vi "Best_n_routine_PN.vi"(3 "fixed n":dbl=0.4, 4 "variable n?":bool=TRUE, 5 "U":dbl[](array[numeric])=[1.9700640366, 2.9544254558, 3.9511341522, 4.988746499, 5.9653548413, 6.955762857, 7.9505145639, 8.9534679688, 9.9841669593, 10.940163718], 6 "E^2":dbl[](array[numeric])=[2.545899323848856, 2.7039683334539926, 2.834095502347166, 2.9505738427182537, 3.0478567682958038, 3.136700737890616, 3.218281943968314, 3.2949717775853564, 3.3680504701927467, 3.4322041581183096]) -> (0 "n":dbl=0.3999859587965401 format="%#_18g", 1 "B":dbl=0.6862228365898919 format="%#_18g", 2 "A":dbl=1.6456605879472355 format="%#_18g")   [LabVIEW 2010]
uses:
  <vilib>/Analysis/7linalg.llb/Solve Linear Equations (single right hand).vi
  <vilib>/Analysis/baseanly.llb/Real A x B.vi
  <vilib>/Analysis/7linalg.llb/Solve Linear Eqs (General).vi
  <vilib>/Analysis/7linalg.llb/Solve Linear Eqs (Gen, single right hand).vi
  <vilib>/Analysis/Matrix/Numeric/Conversions/Array To Matrix - RA2.vi
  <vilib>/Analysis/7linalg.llb/Real Transpose Matrix.vi
  <vilib>/Analysis/baseanly.llb/Real Inverse Matrix.vi
  <vilib>/Analysis/baseanly.llb/A x Vector.vi
  Globals/Dynamic_call_global.ph.vi
  <vilib>/Analysis/NI_AALPro.lvlib
  <vilib>/Analysis/NI_AALBase.lvlib
  <vilib>/Analysis/Matrix/NI_Matrix.lvlib
panel:
  in  "dn":dbl=0.0001
  in  "nmin":dbl=0.2
  in  "nmax":dbl=0.8
  in  "output RMS err?":bool=TRUE
  out "RMS err in U (m/s)":dbl=0.002670941583711803 format="%#_3f"
  out "abs rel. err.":dbl[](array[numeric])=[3.983055063353366e-13, 8.213953245912097e-13, 5.386158518578956e-13] format="%#.6e"
  out "NLR against data":cluster{dbl[], "U":dbl[]}[](graph)=[{[0.1, 0.122, 0.14884, 0.1815848, 0.221533456, 0.27027081632, 0.3297303959104, 0.402271083010688, 0.49077072127303933, 0.598740279953108, 0.7304631415427917, 0.8911650326822058, 1.087221339872291, 1.326410034644195, 1.6182202422659178, 1.9742286955644197, 2.408559008588592, 2.9384419904780823, 3.5848992283832604, 4.3735770586275775, 5.335764011525645, 6.509632094061287, 7.94175115475477, 9.688936408800819, 11.820502418736998, 14.421012950859138, 17.593635800048148, 21.46423567605874, 26.18636752479166, 31.947368380245823], "U"=[1.918859652465371, 1.9414767700229, 1.9659662732253556, 1.992483169800597, 2.021195299980173, 2.052284398853782, 2.0859472466720375, 2.1223969143784562, 2.161864112254325, 2.204598650212778, 2.2508710189851024, 2.3009741022074746, 2.3552250302448847, 2.413967187486141, 2.477572385815227, 2.5464432180161425, 2.6210156060072305, 2.7017615600341864, 2.7891921662862273, 2.8838608218457082, 2.9863667374469767, 3.097358730215403, 3.2175393303929196, 3.34766922804385, 3.488572087886694, 3.6411397627276374, 3.8063379384945, 3.985212246601707, 4.178894882334845, 4.388611771146246]}, {[1.9700640366, 2.9544254558, 3.9511341522, 4.988746499, 5.9653548413, 6.955762857, 7.9505145639, 8.9534679688, 9.9841669593, 10.940163718], "U"=[2.545899323848856, 2.7039683334539926, 2.834095502347166, 2.9505738427182537, 3.0478567682958038, 3.136700737890616, 3.218281943968314, 3.2949717775853564, 3.3680504701927467, 3.4322041581183096]}]
  in  "n0":dbl=1.0
  in  "B0":dbl=2.0
  in  "A0":dbl=10.0
  in  "show iters\ngraphically":bool
  in  "tol.":dbl=1e-12
  in  "max. iter":i32=1000
  in  "retardation":dbl=0.5
  out "Iterations":i32=47
  # "Linearise by Taylor series up to first order."
  # "if variable n is false, then this value is used for n"
  # "for coersion"
  # "r is the retardation parameter 0...1"
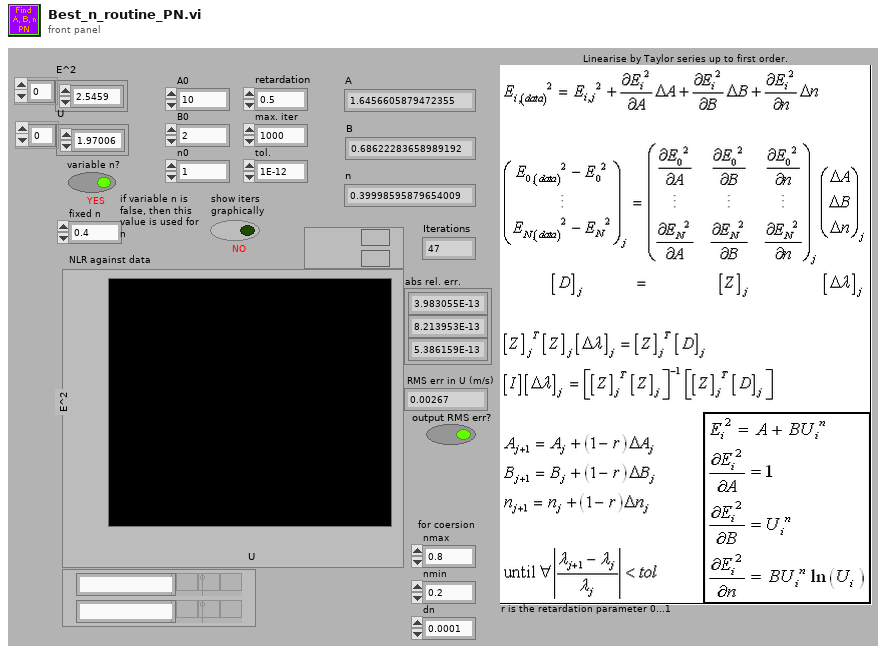
[diagram p1: front panel]
types:
  T1 = typedef "NI_Matrix.lvlib/RealMatrix.ctl" = dbl[][]
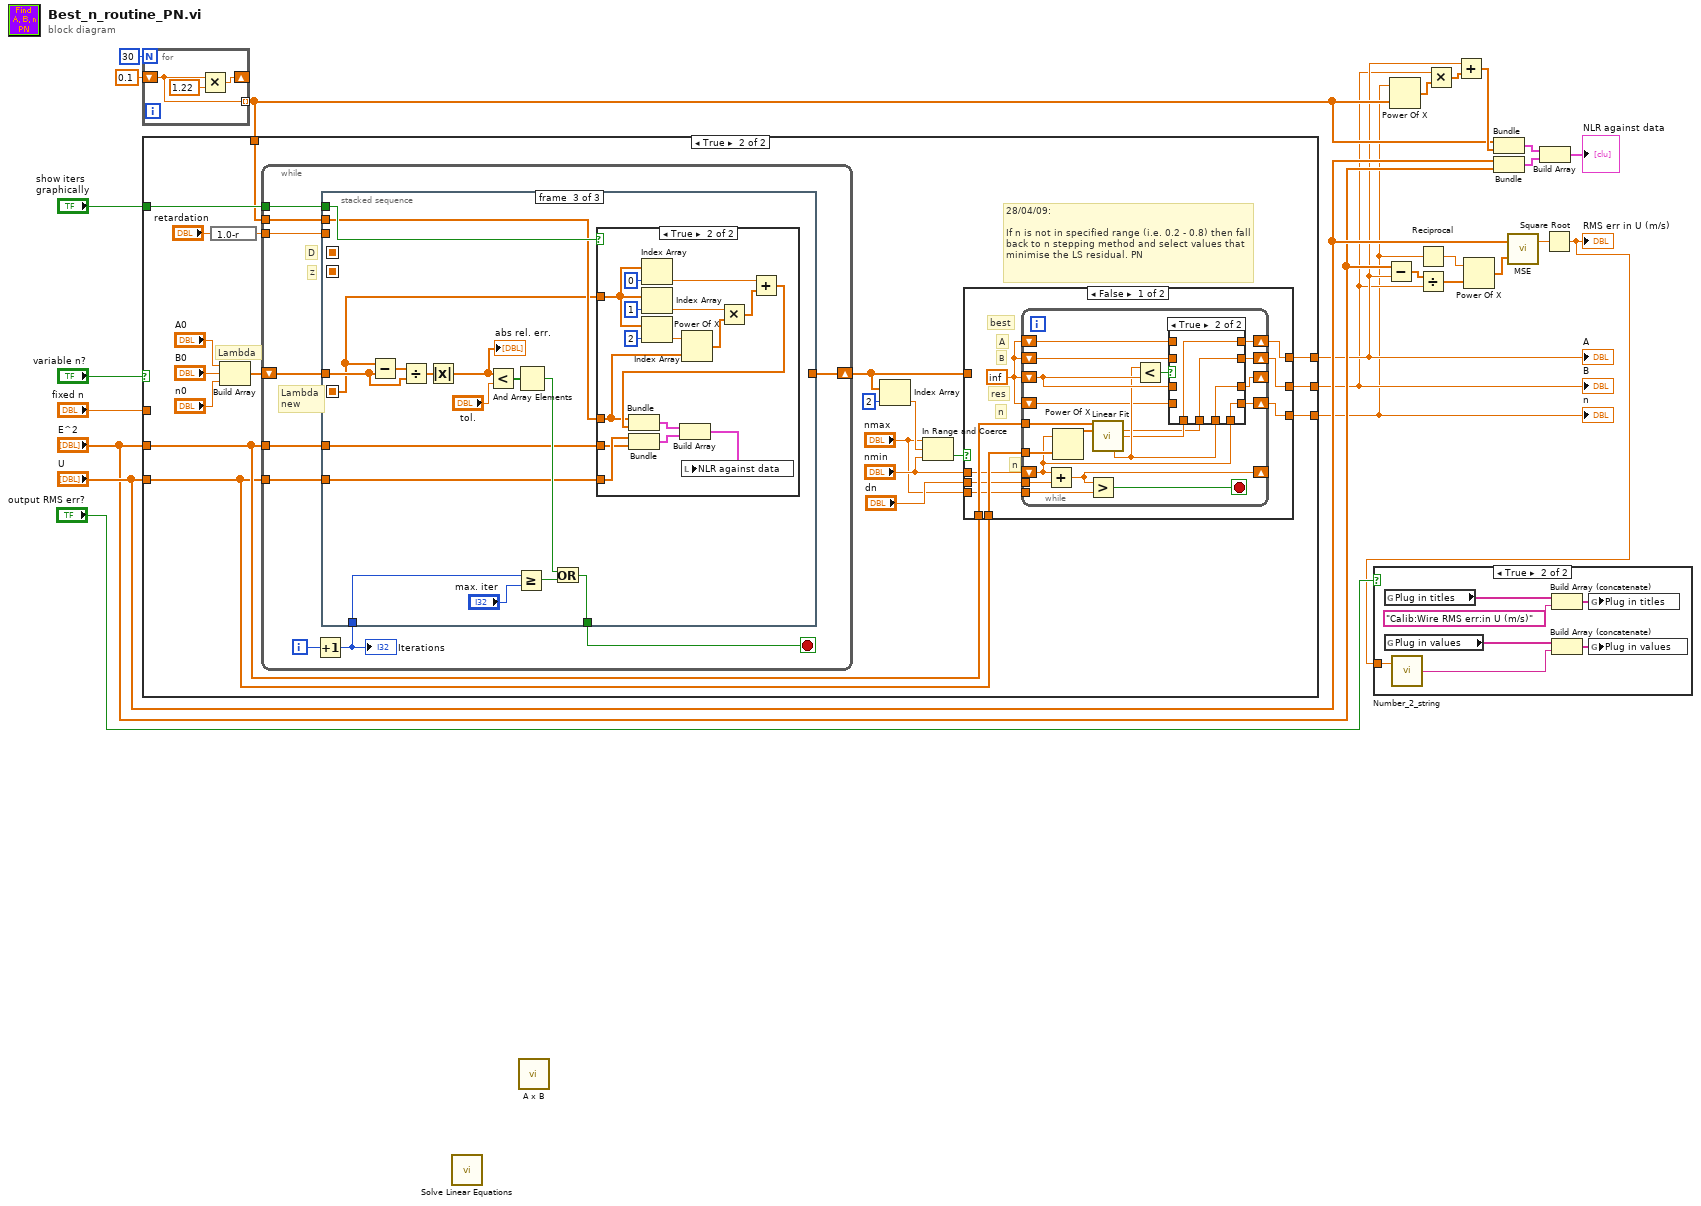
[diagram p0: block diagram]
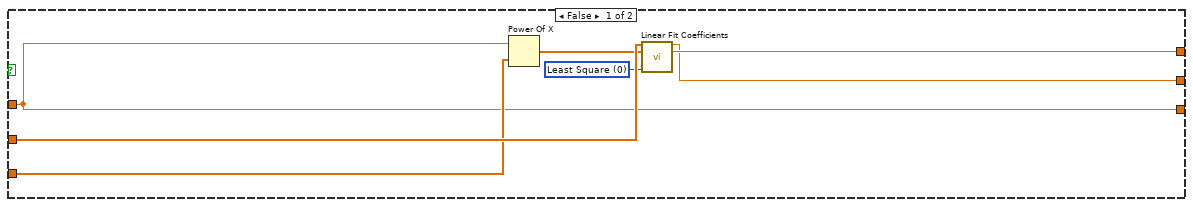
[diagram p3: hidden frame]
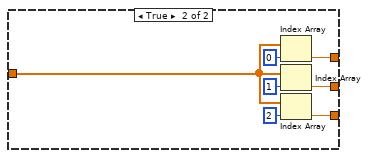
[diagram p5: hidden frame]
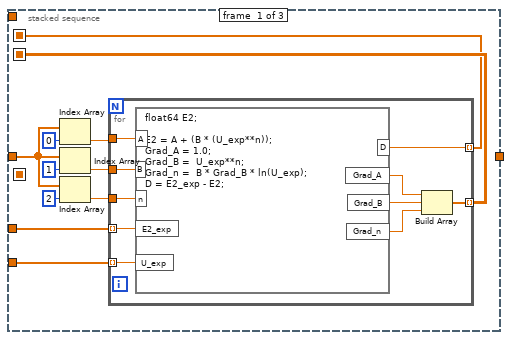
[diagram p6: hidden frame]
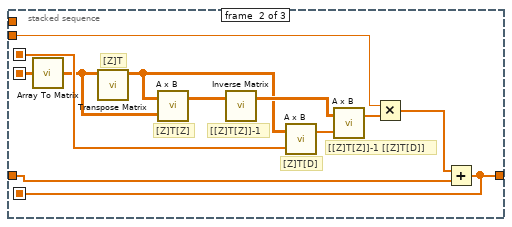
[diagram p7: hidden frame]
diagram:
  n1 = for {
    N: 30 ("dimension size") -> [_]
    shift-right: [w26] -> _
    shift-left: 0.1 ("element") -> [w25]
    tunnel: [w25] -> w13 mode=indexing
    n2 = Multiply(x=w25, y=1.22) -> (x*y=w26:dbl)
  }
  n3 = case shown="True" "variable n?" {
    tunnel: "U" -> [w33 w41]
    tunnel: "show iters\ngraphically" -> [_ w52]
    tunnel: w13 -> [_ w51]
    tunnel: "E^2" -> [w34 w42]
    tunnel: "fixed n" -> [w28 _]
    tunnel: [w30 w37] -> w3
    tunnel: [w29 w36] -> w2
    tunnel: [w28 w35] -> w1
    frame False {
      w31 = u16 0 items=["Least Square", "Least Absolute Residual", "Bisquare"] ("method")
      n4 = Power Of X(1:w33, 2:w28) -> (0:w32:dbl[])
      n5 = call <vilib>:"Linear Fit Coefficients.vi"("Y"=w34, "X"=w32, "method"=w31) -> ("slope"=w29:dbl, "intercept"=w30:dbl)  [unwired: 2 in, 9 out]
    }
    frame True {
      # "28/04/09:\n\nIf n is not in specified range (i.e. 0.2 - 0.8) then fall back to n stepping method and select values that minimise the LS residual. PN"
      # "Lambda"
      n6 = expression code="1.0-r"("retardation") -> (w53:dbl)
      n7 = Build Array("A0", "B0", "n0") -> (w47:dbl[])
      n8 = while {
        tunnel: w42 -> [w108]
        tunnel: w41 -> [w107]
        shift-right: [w106] -> w44
        shift-left: w47 -> [w105]
        tunnel: w53 -> [w103]
        tunnel: w52 -> [w102]
        tunnel: w51 -> [w101]
        i -> [w100]
        stop <- w104 stop-if-true
        # "Lambda\nnew"
        # "D"
        # "Z"
        n9 = Increment(x=w100) -> (x+1=w99:i32)
        "Iterations" <- w99
        n10 = stacked-sequence {
          seq-local: [w116 _ _] -> [_ w137 _]
          seq-local: [w117 _ _] -> [_ w133 _]
          seq-local: [_ w130 _] -> [_ _ w142]
          tunnel: w108 -> [w119 _ w152]
          tunnel: w107 -> [w118 _ w151]
          tunnel: [_ w130 _] -> w106
          tunnel: w105 -> [w110 w131 w157]
          tunnel: [_ _ w154] -> w104
          tunnel: w99 -> [_ _ w145]
          tunnel: w103 -> [_ w135 _]
          tunnel: w102 -> [_ _ w150]
          tunnel: w101 -> [_ _ w149]
          frame #0 {
            n11 = Index Array(array=w110, index=0) -> (element=w112:dbl)
            n12 = Index Array(array=w110, index=1) -> (element=w111:dbl)
            n13 = Index Array(array=w110, index=2) -> (element=w109:dbl)
            n14 = for {
              tunnel: w119 -> [w129] mode=indexing
              tunnel: w118 -> [w128] mode=indexing
              tunnel: [w124] -> w117 mode=indexing
              tunnel: [w123] -> w116 mode=indexing
              tunnel: w112 -> [w122]
              tunnel: w111 -> [w121]
              tunnel: w109 -> [w120]
              n15 = formula code="float64 E2;\n\nE2 = A + (B * (U_exp**n));\nGrad_A = 1.0;\nGrad_B =  U_exp**n;\nGrad_n =  B * Grad_B * ln(U_exp);\nD = E2_exp - E2;"("E2_exp"=w129, "U_exp"=w128, "A"=w122, "B"=w121, "n"=w120) -> ("D"=w123:dbl, "Grad_A"=w127:dbl, "Grad_B"=w126:dbl, "Grad_n"=w125:dbl)
              n16 = Build Array(w127, w126, w125) -> (w124:dbl[])
            }
          }
          frame #1 {
            # "[[Z]T[Z]]-1 [[Z]T[D]]"
            # "[Z]T[D]"
            # "[[Z]T[Z]]-1"
            # "[Z]T[Z]"
            # "[Z]T"
            n17 = call-poly <vilib>:"Array To Matrix.vi"("Real 2D Array"=w133) -> ("Real Matrix"=w134:T1)
            n18 = call-poly <vilib>:"Transpose Matrix.vi"("Input Matrix"=w134) -> ("Matrix Transpose"=w138:T1)  [unwired: 10 out]
            n19 = call-poly <vilib>:"A x B.vi"("B"=w134, "A"=w138) -> ("A x B"=w141:T1)  [unwired: 1 out]
            n20 = call-poly <vilib>:"Inverse Matrix.vi"("Input Matrix"=w141) -> ("Inverse Matrix"=w140:T1)  [unwired: 1 in, 1 out]
            n21 = call-poly <vilib>:"A x B.vi"("Vector"=w137, "A"=w138) -> ("A x Vector"=w139:dbl[])  [unwired: 1 out]
            n22 = call-poly <vilib>:"A x B.vi"("Vector"=w139, "A"=w140) -> ("A x Vector"=w136:dbl[])  [unwired: 1 out]
            n23 = Multiply(x=w135, y=w136) -> (x*y=w132:dbl[])
            n24 = Add(x=w132, y=w131) -> (x+y=w130:dbl[])
          }
          frame #2 {
            n25 = Subtract(x=w142, y=w157) -> (x-y=w146:dbl[])
            n26 = Divide(x=w146, y=w157) -> (x/y=w144:dbl[])
            n27 = Absolute Value(x=w144) -> (abs(x)=w143:dbl[])
            "abs rel. err." <- w143
            n28 = Less?(x=w143, y="tol.") -> (x < y?=w147:bool[])
            n29 = Greater Or Equal?(x=w145, y="max. iter") -> (x >= y?=w155:bool)
            n30 = And Array Elements(Boolean array=w147) -> (logical AND=w153:bool)
            n31 = Or(x=w153, y=w155) -> (x .or. y?=w154:bool)
            n32 = case shown="True" w150 {
              tunnel: w152 -> [_ w167]
              tunnel: w151 -> [_ w168]
              tunnel: w149 -> [_ w166]
              tunnel: w142 -> [_ w162]
              frame False {
              }
              frame True {
                n33 = Bundle("U"=w168, "E^2"=w167) -> (w171:cluster{"U":dbl[], "E^2":dbl[]})  [unwired: 1 out]
                n34 = Index Array(array=w162, index=0) -> (element=w161:dbl)
                n35 = Index Array(array=w162, index=1) -> (element=w160:dbl)
                n36 = Index Array(array=w162, index=2) -> (element=w159:dbl)
                n37 = Power Of X(1:w166, 2:w159) -> (0:w173:dbl[])
                n38 = Multiply(x=w160, y=w173) -> (x*y=w172:dbl[])
                n39 = Add(x=w161, y=w172) -> (x+y=w169:dbl[])
                n40 = Bundle(w166, w169) -> (w170:cluster{dbl[], dbl[]})  [unwired: 1 out]
                n41 = Build Array(w170, w171) -> (w158:cluster{"U":dbl[], "E^2":dbl[]}[])
                n42 = local write "NLR against data"(w158) -> ()
              }
            }
          }
        }
      }
      n43 = Index Array(array=w44, index=2) -> (element=w45:dbl)
      n44 = In Range and Coerce(upper limit="nmax", x=w45, lower limit="nmin") -> (In Range?=w43:bool)  [unwired: 1 out]
      n45 = case shown="False" w43 {
        tunnel: w44 -> [_ w95]
        tunnel: w42 -> [w63 _]
        tunnel: w41 -> [w62 _]
        tunnel: "nmin" -> [w61 _]
        tunnel: "dn" -> [w60 _]
        tunnel: "nmax" -> [w59 _]
        tunnel: [w58 w94] -> w37
        tunnel: [w57 w93] -> w36
        tunnel: [w55 w92] -> w35
        frame False {
          w56 = inf
          # "best"
          # "n"
          # "n"
          # "res"
          # "B"
          # "A"
          n46 = while {
            tunnel: w62 -> [w83]
            tunnel: w63 -> [w81]
            shift-right: [w78] -> _
            shift-left: w61 -> [w64]
            tunnel: w60 -> [w80]
            tunnel: w59 -> [w79]
            shift-right: [w72] -> w57
            shift-left: w56 -> [w73]
            shift-right: [w74] -> w58
            shift-left: w56 -> [w75]
            shift-right: [w70] -> _
            shift-left: w56 -> [w71]
            shift-right: [w66] -> w55
            shift-left: w56 -> [w65]
            stop <- w77 stop-if-true
            n47 = Add(x=w64, y=w80) -> (x+y=w78:dbl)
            n48 = Power Of X(1:w83, 2:w64) -> (0:w82:dbl[])
            n49 = Greater?(x=w78, y=w79) -> (0:w77:bool)
            n50 = call <vilib>:"Linear Fit.vi"("Y"=w81, "X"=w82) -> ("slope"=w67:dbl, "intercept"=w68:dbl, "residue"=w69:dbl)  [unwired: 4 in, 7 out]
            n51 = Less?(x=w69, y=w71) -> (x < y?=w76:bool)
            n52 = case shown="True" w76 {
              tunnel: [w87 w90] -> w74
              tunnel: w75 -> [w87 _]
              tunnel: w73 -> [w86 _]
              tunnel: [w86 w89] -> w72
              tunnel: w71 -> [w85 _]
              tunnel: [w85 w91] -> w70
              tunnel: w69 -> [_ w91]
              tunnel: w68 -> [_ w90]
              tunnel: w67 -> [_ w89]
              tunnel: w64 -> [_ w88]
              tunnel: [w84 w88] -> w66
              tunnel: w65 -> [w84 _]
              frame False {
              }
              frame True {
              }
            }
          }
        }
        frame True {
          n53 = Index Array(array=w95, index=0) -> (element=w94:dbl)
          n54 = Index Array(array=w95, index=1) -> (element=w93:dbl)
          n55 = Index Array(array=w95, index=2) -> (element=w92:dbl)
        }
      }
    }
  }
  "n" <- w1
  "B" <- w2
  "A" <- w3
  n56 = call-poly <vilib>:"Solve Linear Equations.vi"() -> ()  [unwired: 3 in, 2 out]
  n57 = call-poly <vilib>:"A x B.vi"() -> ()  [unwired: 2 in, 2 out]
  n58 = Subtract(x="E^2", y=w3) -> (x-y=w10:dbl[])
  n59 = Power Of X(1:w13, 2:w1) -> (0:w16:dbl[])
  n60 = Reciprocal(x=w1) -> (1/x=w9:dbl)
  n61 = Divide(x=w10, y=w2) -> (x/y=w8:dbl[])
  n62 = Multiply(x=w2, y=w16) -> (x*y=w17:dbl[])
  n63 = Add(x=w3, y=w17) -> (x+y=w15:dbl[])
  n64 = Power Of X(1:w8, 2:w9) -> (0:w7:dbl[])
  n65 = Bundle(w13, w15) -> (w19:cluster{dbl[], dbl[]})  [unwired: 1 out]
  n66 = Bundle("U"="U", "E^2"="E^2") -> (w18:cluster{"U":dbl[], "E^2":dbl[]})  [unwired: 1 out]
  n67 = call <vilib>:"MSE.vi"("X Values"=w7, "Y Values"="U") -> ("mse"=w6:dbl)  [unwired: 1 out]
  n68 = Build Array(w19, w18) -> (→"NLR against data":cluster{"U":dbl[], "E^2":dbl[]}[])
  n69 = Square Root(x=w6) -> (sqrt(x)=w4:dbl)
  "RMS err in U (m/s)" <- w4
  n70 = case shown="True" "output RMS err?" {
    tunnel: w4 -> [_ w174]
    frame False {
    }
    frame True {
      n71 = global read "Dynamic_call_global.ph.vi" "Plug in titles"() -> (w178:string[])
      n72 = global read "Dynamic_call_global.ph.vi" "Plug in values"() -> (w177:string[])
      n73 = call "Number_2_string.vi"("number"=w174) -> ("String"=w175:string)  [unwired: 1 in]
      n74 = Build Array (concatenate)(w178, "Calib:Wire RMS err:in U (m/s)") -> (w180:string[])
      n75 = Build Array (concatenate)(w177, w175) -> (w179:string[])
      n76 = global write "Dynamic_call_global.ph.vi" "Plug in titles"(w180) -> ()
      n77 = global write "Dynamic_call_global.ph.vi" "Plug in values"(w179) -> ()
    }
  }
